vi "Set To Complete Status.vi"(8 "error in (no error)":errorcluster, 11 "Operation Complete Caller in":refnum<class "Operation Complete Caller.lvclass">) -> (0 "error out":errorcluster, 3 "Operation Complete Caller out":refnum<class "Operation Complete Caller.lvclass">)   [LabVIEW 2022 SP3, in "Operation Complete Caller.lvclass"]
uses:
  Operation Complete Caller.lvclass
  Operation Complete Caller.lvclass/Operation Complete Caller.ctl
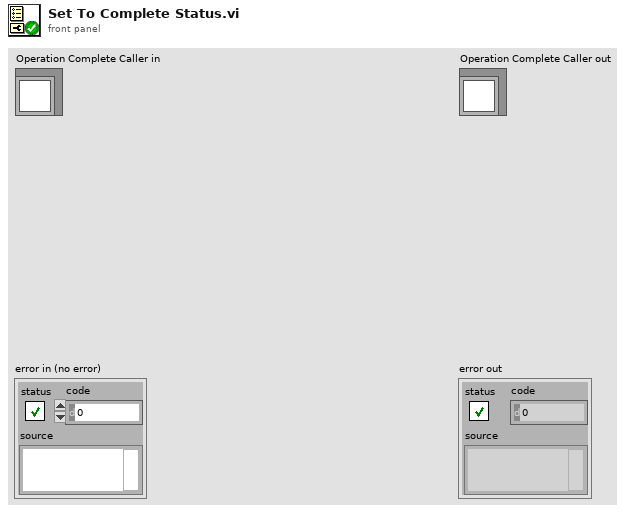
[diagram p1: front panel]
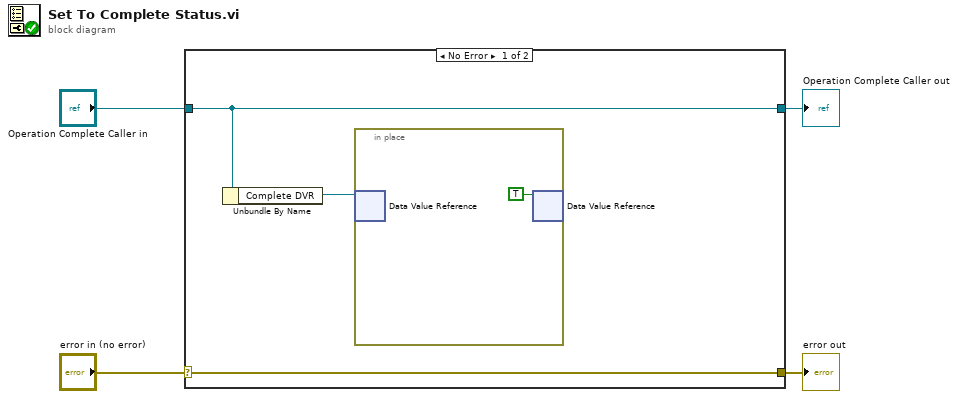
[diagram p0: block diagram]
diagram:
  n1 = case shown="No Error" "error in (no error)" {
    selector: "error in (no error)" -> [w7 w10]
    tunnel: [w7 w10] -> w3
    tunnel: [w6 w9] -> w1
    tunnel: "Operation Complete Caller in" -> [w6 w9]
    frame No Error {
      n2 = Unbundle By Name(w6) -> ("Complete DVR"=w5:refnum<data-value>)
      n3 = in-place {
        n4 = in-place-dvr #1(w5) -> ()  [unwired: 2 out]
        n5 = in-place-dvr #1(TRUE ("data value")) -> ()  [unwired: 2 out]
      }
    }
    frame Error {
    }
  }
  "error out" <- w3
  "Operation Complete Caller out" <- w1
